vi "CTR-Compute Ticks.vi"(0 "Sampling Rate (Hz)":dbl, 1 "Delay (ms)":dbl, 3 "pulse duration (ms)":dbl=0.25, 5 "Npts":i32, 11 "error in (no error)":errorcluster) -> (4 "Hi ticks":u32=5, 6 "Low ticks":u32=4995 max=1, 8 "Idle state":i32(ring)=10214 caption="Idle State" items=["High"=10192, "Low"=10214], 10 "Delay ticks":u32, 15 "error out":errorcluster)   [LabVIEW 2020]
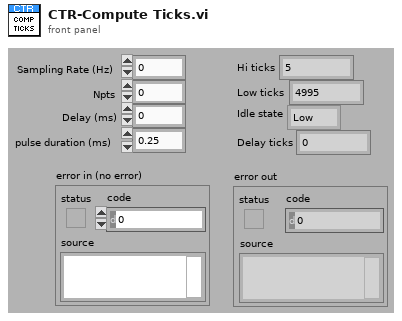
[diagram p1: front panel]
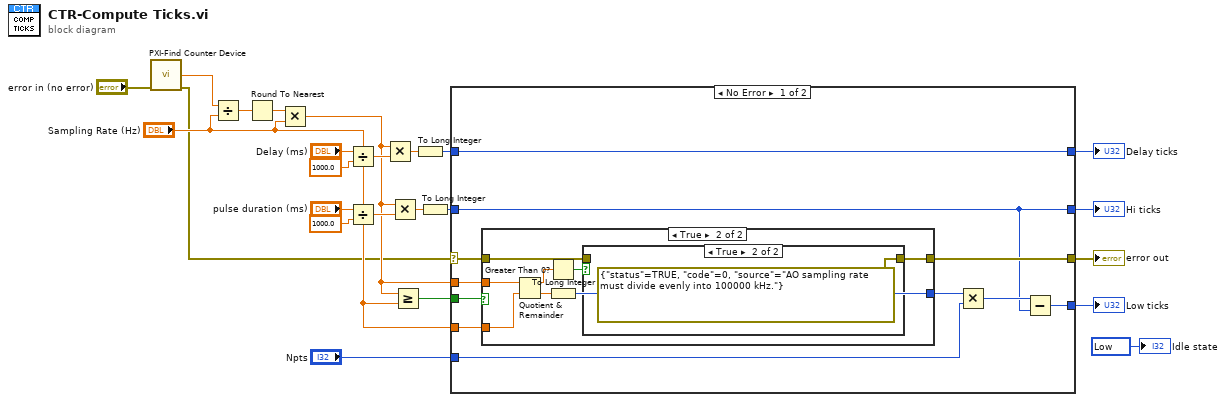
[diagram p0: block diagram]
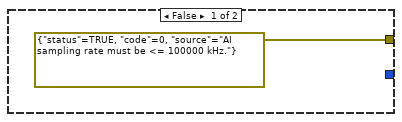
[diagram p2: hidden frame]
diagram:
  w1 = 10214 items=["High"=10192, "Low"=10214] ("Idle state")
  n1 = call "PXI-Find Counter Device.vi"("error in (no error)"="error in (no error)") -> ("Clock Rate"=w7:dbl, "error out"=w5:errorcluster)  [unwired: 10 in, 3 out]
  n2 = Divide(x=w7, y="Sampling Rate (Hz)") -> (x/y=w11:dbl)
  n3 = Round To Nearest(number=w11) -> (nearest integer value=w10:dbl)
  n4 = Multiply(x=w10, y="Sampling Rate (Hz)") -> (x*y=w8:dbl)
  n5 = Divide(x="Delay (ms)", y=1000.0) -> (x/y=w21:dbl)
  n6 = Divide(x="pulse duration (ms)", y=1000.0) -> (x/y=w16:dbl)
  n7 = Multiply(x=w8, y=w21) -> (x*y=w23:dbl)
  n8 = Multiply(x=w8, y=w16) -> (x*y=w24:dbl)
  n9 = Greater Or Equal?(x=w8, y="Sampling Rate (Hz)") -> (x >= y?=w18:bool)
  n10 = To Long Integer(number=w23) -> (32bit integer=w14:i32)
  n11 = To Long Integer(number=w24) -> (32bit integer=w13:i32)
  n12 = case shown="No Error" w5 {
    selector: w5 -> [w30 w47]
    tunnel: w18 -> [w35 _]
    tunnel: "Npts" -> [w34 _]
    tunnel: w14 -> [w27 _]
    tunnel: w13 -> [w26 _]
    tunnel: [w33 w47] -> w12
    tunnel: "Sampling Rate (Hz)" -> [w32 _]
    tunnel: w8 -> [w31 _]
    tunnel: [w27 _] -> w4
    tunnel: [w26 _] -> w3
    tunnel: [w25 _] -> w2
    frame No Error {
      n13 = case shown="True" w35 {
        tunnel: w31 -> [_ w44]
        tunnel: w32 -> [_ w43]
        tunnel: [_ w41] -> w28
        tunnel: w30 -> [_ w38]
        tunnel: [errorcluster {"status"=TRUE, "code"=0, "source"="AI sampling rate must be <= 100000 kHz."} ("error in (no error)") w37] -> w33
        frame False {
        }
        frame True {
          n14 = Quotient & Remainder(x=w44, y=w43) -> (x-y*floor(x/y)=w39:dbl, floor(x/y)=w42:dbl)
          n15 = Greater Than 0?(x=w39) -> (x > 0?=w40:bool)
          n16 = To Long Integer(number=w42) -> (32bit integer=w41:i32)
          n17 = case shown="True" w40 {
            tunnel: w38 -> [w45 _]
            tunnel: [w45 errorcluster {"status"=TRUE, "code"=0, "source"="AO sampling rate must divide evenly into 100000 kHz."} ("error in (no error)")] -> w37
            frame False {
            }
            frame True {
            }
          }
        }
      }
      n18 = Multiply(x=w28, y=w34) -> (x*y=w29:i32)
      n19 = Subtract(x=w29, y=w26) -> (x-y=w25:i32)
    }
    frame Error {
    }
  }
  "error out" <- w12
  "Hi ticks" <- w3
  "Low ticks" <- w2
  "Delay ticks" <- w4
  "Idle state" <- w1
